vi "FTW-Container-Equality.vi"(0 "FTW-Container In":refnum<class "FTW-Container.lvclass">, 5 "Other Container":refnum<class "FTW-Container.lvclass">, 11 "error in":errorcluster) -> (4 "FTW-Container Out":refnum<class "FTW-Container.lvclass">, 8 "Equal":bool, 15 "error out":errorcluster)   [LabVIEW 2015, in "FTW-Container.lvclass"]
uses:
  FTW-Container.lvclass
  FTW-Container-Type.ctl
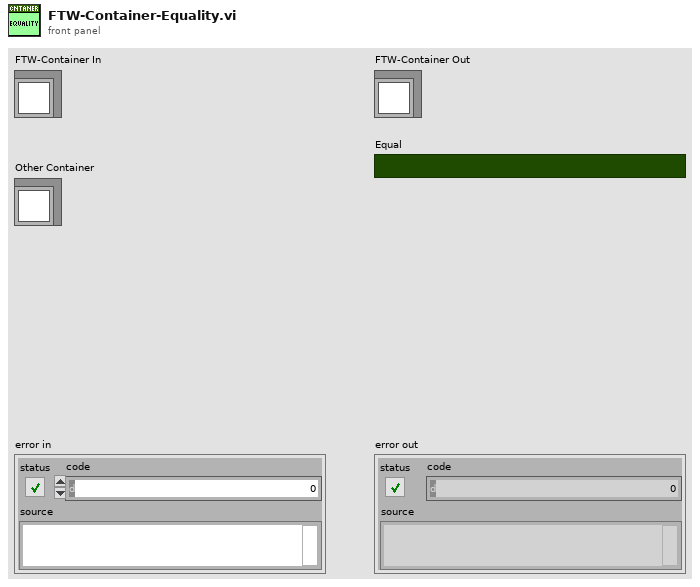
[diagram p1: front panel]
types:
  T1 = typedef "FTW-Container.lvclass/FTW-Container-Type.ctl" = enum8{"invalid", "String", "Integer", "Real", "Object", "Array", "Boolean", "null"}
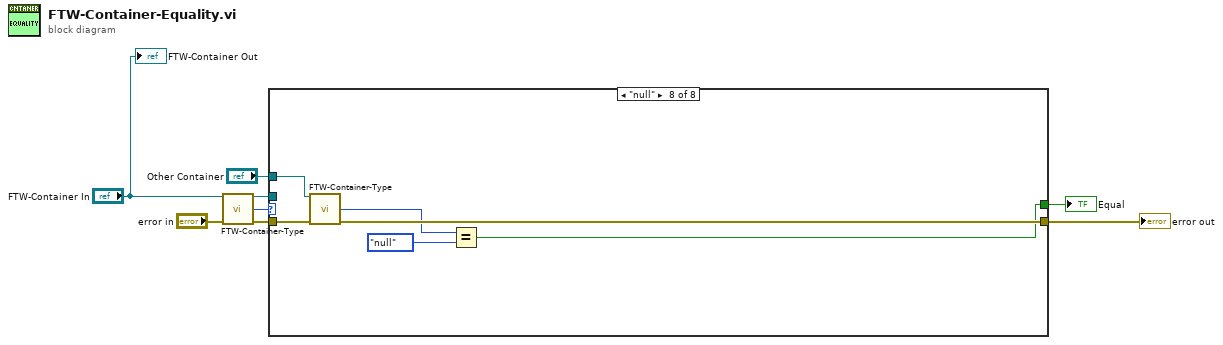
[diagram p0: block diagram]
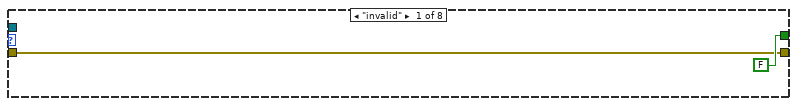
[diagram p2: hidden frame]
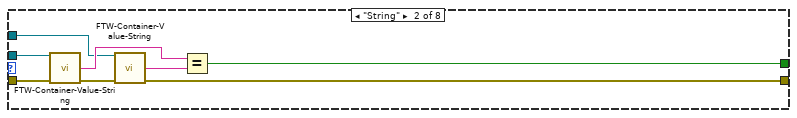
[diagram p3: hidden frame]
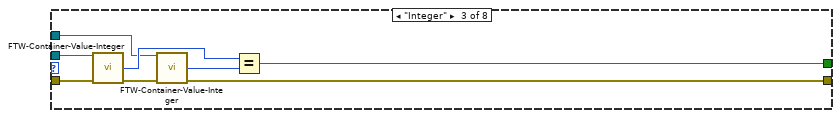
[diagram p4: hidden frame]
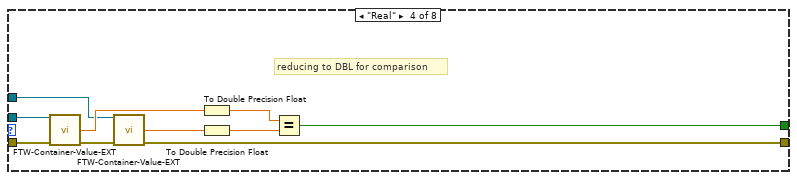
[diagram p5: hidden frame]
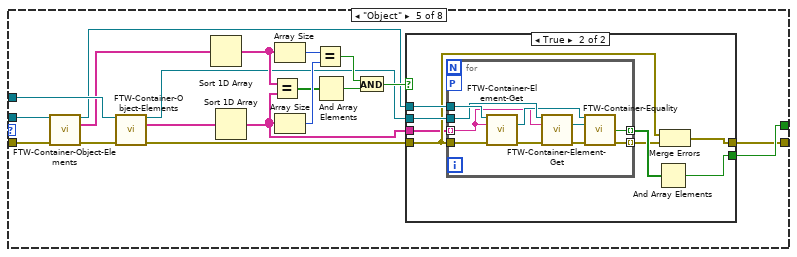
[diagram p6: hidden frame]
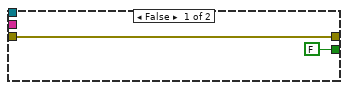
[diagram p7: hidden frame]
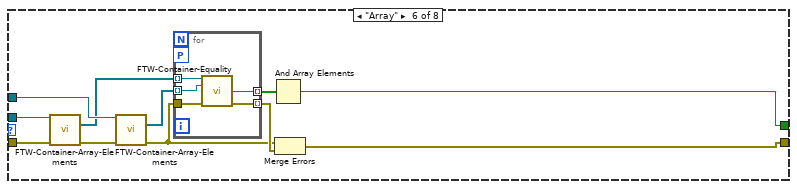
[diagram p8: hidden frame]
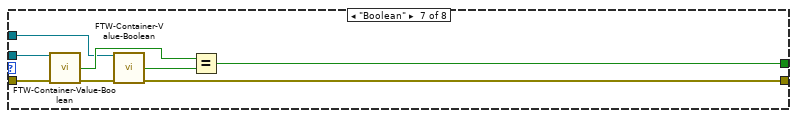
[diagram p9: hidden frame]
diagram:
  n1 = call "FTW-Container-Type.vi"("FTW-Container In"="FTW-Container In", "error in"="error in") -> ("FTW-Container Out"=w4:refnum<class "FTW-Container.lvclass">, "Type"=w7:T1, "error out"=w3:errorcluster)  [unwired: 11 in]
  n2 = case shown="\"null\"" w7 {
    tunnel: "Other Container" -> [_ w15 w23 w33 w54 w84 w96 w103]
    tunnel: [FALSE w18 w26 w36 w52 w80 w99 w100] -> w5
    tunnel: w4 -> [_ w17 w25 w35 w55 w85 w98 _]
    tunnel: w3 -> [w9 w13 w21 w31 w53 w83 w94 w105]
    tunnel: [w9 w11 w19 w27 w51 w78 w92 w104] -> w1
    frame "invalid" {
    }
    frame "String" {
      n3 = call "FTW-Container-Value-String.vi"("JSON"=w17, "error in"=w13) -> ("Value"=w16:string, "error out"=w12:errorcluster)  [unwired: 11 in, 1 out]
      n4 = call "FTW-Container-Value-String.vi"("JSON"=w15, "error in"=w12) -> ("Value"=w14:string, "error out"=w11:errorcluster)  [unwired: 11 in, 1 out]
      n5 = Equal?(x=w16, y=w14) -> (x = y?=w18:bool)
    }
    frame "Integer" {
      n6 = call "FTW-Container-Value-Integer.vi"("JSON"=w25, "error in"=w21) -> ("Value"=w24:i64, "error out"=w20:errorcluster)  [unwired: 11 in, 1 out]
      n7 = call "FTW-Container-Value-Integer.vi"("JSON"=w23, "error in"=w20) -> ("Value"=w22:i64, "error out"=w19:errorcluster)  [unwired: 11 in, 1 out]
      n8 = Equal?(x=w24, y=w22) -> (x = y?=w26:bool)
    }
    frame "Real" {
      # "reducing to DBL for comparison"
      n9 = call "FTW-Container-Value-EXT.vi"("JSON"=w35, "error in"=w31) -> ("Value"=w34:ext, "error out"=w28:errorcluster)  [unwired: 11 in, 1 out]
      n10 = call "FTW-Container-Value-EXT.vi"("JSON"=w33, "error in"=w28) -> ("Value"=w32:ext, "error out"=w27:errorcluster)  [unwired: 11 in, 1 out]
      n11 = To Double Precision Float(number=w34) -> (double precision float=w29:dbl)
      n12 = To Double Precision Float(number=w32) -> (double precision float=w30:dbl)
      n13 = Equal?(x=w29, y=w30) -> (x = y?=w36:bool)
    }
    frame "Object" {
      n14 = call "FTW-Container-Object-Elements.vi"("FTW-Container In"=w55, "error in"=w53) -> ("FTW-Container Out"=w39:refnum<class "FTW-Container.lvclass">, "Names"=w49:string[], "error out"=w38:errorcluster)  [unwired: 10 in, 1 out]
      n15 = call "FTW-Container-Object-Elements.vi"("FTW-Container In"=w54, "error in"=w38) -> ("FTW-Container Out"=w40:refnum<class "FTW-Container.lvclass">, "Names"=w50:string[], "error out"=w37:errorcluster)  [unwired: 10 in, 1 out]
      n16 = Sort 1D Array(array=w49) -> (sorted array=w46:string[])
      n17 = Sort 1D Array(array=w50) -> (sorted array=w41:string[])
      n18 = Equal?(x=w46, y=w41) -> (x = y?=w44:bool[])
      n19 = Array Size(array=w46) -> (size(s)=w48:i32)
      n20 = Array Size(array=w41) -> (size(s)=w47:i32)
      n21 = Equal?(x=w48, y=w47) -> (x = y?=w45:bool)
      n22 = And Array Elements(Boolean array=w44) -> (logical AND=w43:bool)
      n23 = And(x=w45, y=w43) -> (x .and. y?=w42:bool)
      n24 = case shown="True" w42 {
        tunnel: w39 -> [_ w64]
        tunnel: w40 -> [_ w63]
        tunnel: [FALSE w62] -> w52
        tunnel: [w56 w60] -> w51
        tunnel: w37 -> [w56 w59]
        tunnel: w41 -> [_ w58]
        frame False {
        }
        frame True {
          n25 = for {
            tunnel: [w75] -> w65 mode=indexing
            tunnel: w64 -> [w74]
            tunnel: w59 -> [w67]
            tunnel: w63 -> [w73]
            tunnel: [w72] -> w61 mode=indexing
            workers-P: _ -> [_]
            tunnel: w58 -> [w69] mode=indexing
            n26 = call "FTW-Container-Element-Get.vi"("FTW-Container In"=w74, "Element Name"=w69, "error in"=w67) -> ("Element Out"=w71:refnum<class "FTW-Container.lvclass">, "error out"=w66:errorcluster)  [unwired: 9 in, 2 out]
            n27 = call "FTW-Container-Element-Get.vi"("FTW-Container In"=w73, "Element Name"=w69, "error in"=w66) -> ("Element Out"=w70:refnum<class "FTW-Container.lvclass">, "error out"=w68:errorcluster)  [unwired: 9 in, 2 out]
            n28 = call "FTW-Container-Equality.vi"("FTW-Container In"=w71, "Other Container"=w70, "error in"=w68) -> ("Equal"=w75:bool, "error out"=w72:errorcluster)  [unwired: 10 in, 1 out]
          }
          n29 = And Array Elements(Boolean array=w65) -> (logical AND=w62:bool)
          n30 = Merge Errors(w59, w61) -> (w60:errorcluster)
        }
      }
    }
    frame "Array" {
      n31 = call "FTW-Container-Array-Elements.vi"("FTW-Container In"=w85, "error in"=w83) -> ("Array Elements"=w82:refnum<class "FTW-Container.lvclass">[], "error out"=w77:errorcluster)  [unwired: 11 in, 1 out]
      n32 = call "FTW-Container-Array-Elements.vi"("FTW-Container In"=w84, "error in"=w77) -> ("Array Elements"=w81:refnum<class "FTW-Container.lvclass">[], "error out"=w76:errorcluster)  [unwired: 11 in, 1 out]
      n33 = for {
        tunnel: [w91] -> w86 mode=indexing
        tunnel: w82 -> [w90] mode=indexing
        tunnel: w76 -> [w89]
        tunnel: w81 -> [w88] mode=indexing
        tunnel: [w87] -> w79 mode=indexing
        workers-P: _ -> [_]
        n34 = call "FTW-Container-Equality.vi"("FTW-Container In"=w90, "Other Container"=w88, "error in"=w89) -> ("Equal"=w91:bool, "error out"=w87:errorcluster)  [unwired: 10 in, 1 out]
      }
      n35 = And Array Elements(Boolean array=w86) -> (logical AND=w80:bool)
      n36 = Merge Errors(w76, w79) -> (w78:errorcluster)
    }
    frame "Boolean" {
      n37 = call "FTW-Container-Value-Boolean.vi"("FTW-Container In"=w98, "error in"=w94) -> ("Value"=w97:bool, "error out"=w93:errorcluster)  [unwired: 11 in, 1 out]
      n38 = call "FTW-Container-Value-Boolean.vi"("FTW-Container In"=w96, "error in"=w93) -> ("Value"=w95:bool, "error out"=w92:errorcluster)  [unwired: 11 in, 1 out]
      n39 = Equal?(x=w97, y=w95) -> (x = y?=w99:bool)
    }
    frame "null" {
      n40 = call "FTW-Container-Type.vi"("FTW-Container In"=w103, "error in"=w105) -> ("Type"=w102:T1, "error out"=w104:errorcluster)  [unwired: 11 in, 1 out]
      n41 = Equal?(x=w102, y=FTW-Container-Type."null" ("x")) -> (x = y?=w100:bool)
    }
  }
  "error out" <- w1
  "Equal" <- w5
  "FTW-Container Out" <- "FTW-Container In"
